vi "Start Polling.vi"(8 "error in (no error)":errorcluster, 11 "OOQMH in":refnum<class "OOQMH.lvclass">) -> (0 "error out":errorcluster, 3 "OOQMH out":refnum<class "OOQMH.lvclass">)   [LabVIEW 2024, in "OOQMH.lvlib" / "OOQMH.lvclass"]
uses:
  OOQMH.lvclass
  OOQMH.lvclass/OOQMH.ctl
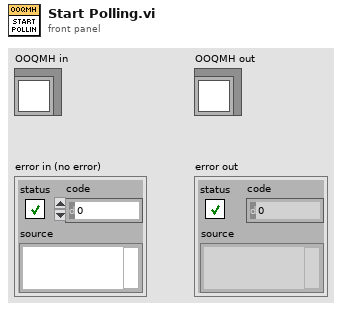
[diagram p1: front panel]
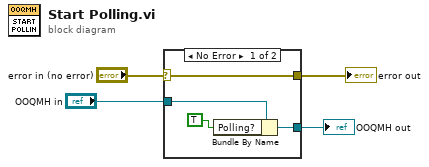
[diagram p0: block diagram]
diagram:
  n1 = case shown="No Error" "error in (no error)" {
    selector: "error in (no error)" -> [w8 w10]
    tunnel: [w8 w10] -> w3
    tunnel: [w5 w9] -> w1
    tunnel: "OOQMH in" -> [w7 w9]
    frame No Error {
      n2 = Bundle By Name(cluster=w7, "Polling?"=TRUE ("Poll?")) -> (w5:refnum<class "OOQMH.lvclass">)
    }
    frame Error {
    }
  }
  "error out" <- w3
  "OOQMH out" <- w1
